vi "Rename.vi"(6 "timeout (ms)":i32=30000, 7 "must be atomic":bool, 8 "error in":errorcluster, 9 "new remote path":string, 10 "old remote path":string, 11 "session in":refnum<class "Session.lvclass">) -> (0 "error out":errorcluster, 3 "session out":refnum<class "Session.lvclass">)   [LabVIEW 2020, in "NI_SFTP.lvlib"]
doc: "Renames a remote file or directory."
uses:
  <vilib>/net/SFTP/NI_SFTP.lvlib
  <vilib>/net/SFTP/Session/Session.lvclass
  <vilib>/net/SFTP/API/Support/Command/SSH_FXP_RENAME/Input.ctl
  <vilib>/Utility/Deadline/NI_Deadline.lvlib
  <vilib>/net/SFTP/API/Support/Command/SSH_FXP_RENAME/SSH_FXP_RENAME.lvclass
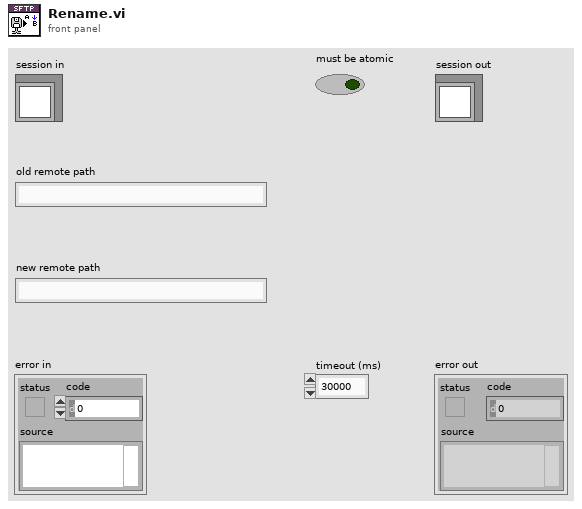
[diagram p1: front panel]
types:
  T1 = typedef "NI_SFTP.lvlib/SSH_FXP_RENAME.lvclass/Input.ctl" = cluster{"old path":string, "new path":string}
  T2 = typedef "NI_Deadline.lvlib/Deadline.ctl" = cluster{"mode":T3, "deadline (ms)":u32}
  T3 = typedef "NI_Deadline.lvlib/Mode.ctl" = enum16{"Relative", "Use deadline", "Wait forever", "Nonblocking", "N/A"}
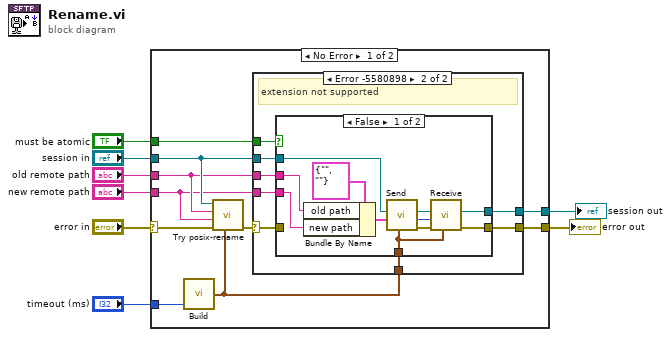
[diagram p0: block diagram]
diagram:
  n1 = case shown="No Error" "error in" {
    selector: "error in" -> [w11 w43]
    tunnel: [w16 w43] -> w6
    tunnel: [w17 w42] -> w1
    tunnel: "session in" -> [w15 w42]
    tunnel: "timeout (ms)" -> [w18 _]
    tunnel: "old remote path" -> [w14 _]
    tunnel: "new remote path" -> [w13 _]
    tunnel: "must be atomic" -> [w9 _]
    frame No Error {
      n2 = call <vilib>:"Build.vi"("timeout (ms)"=w18) -> ("Deadline out"=w12:T2)  [unwired: 2 in]
      n3 = call <vilib>:"Try posix-rename.vi"("Deadline in"=w12, "error in (no error)"=w11, "to"=w13, "from"=w14, "session in"=w15) -> ("error out"=w10:errorcluster)  [unwired: 5 in, 1 out]
      n4 = case shown="Error -5580898" w10 {
        selector: w10 -> [w19 w21]
        tunnel: [w20 w28] -> w17
        tunnel: w15 -> [w20 w27]
        tunnel: [w19 w26] -> w16
        tunnel: w12 -> [_ w25]
        tunnel: w14 -> [_ w24]
        tunnel: w13 -> [_ w23]
        tunnel: w9 -> [_ w22]
        frame #0 {
        }
        frame #1 {
          # "extension not supported"
          n5 = case shown="False" w22 {
            tunnel: [w29 w40] -> w28
            tunnel: w27 -> [w35 w40]
            tunnel: [w37 w41] -> w26
            tunnel: w25 -> [w36 _]
            tunnel: w24 -> [w32 _]
            tunnel: w23 -> [w33 _]
            tunnel: w21 -> [_ w41]
            frame False {
              n6 = Bundle By Name(cluster=T1 {"old path"="", "new path"=""} ("input"), "old path"=w32, "new path"=w33) -> (w31:T1)
              n7 = call <vilib>:"Send.vi"("deadline"=w36, "input"=w31, "session in"=w35) -> ("error out"=w38:errorcluster, "request id"=w30:u32, "session out"=w39:refnum<class "Session.lvclass">)  [unwired: 5 in, 1 out]
              n8 = call <vilib>:"Receive.vi"("deadline"=w36, "error in (no error)"=w38, "request id"=w30, "session in"=w39) -> ("error out"=w37:errorcluster, "session out"=w29:refnum<class "Session.lvclass">)  [unwired: 4 in, 2 out]
            }
            frame True {
            }
          }
        }
      }
    }
    frame Error {
    }
  }
  "error out" <- w6
  "session out" <- w1
